vi "Model Initial Values - Model On Delete Action.vi"(6 "All deleted Refs":T1[](array[typedef]) format="%.0x", 8 "error in (no error)":errorcluster, 11 "Item Ref in":T1 format="%.0x") -> (0 "error out":errorcluster, 3 "Item Ref out":T1 format="%.0x")   [LabVIEW 2011, in "Model Initial Values Custom Device.lvlib"]
uses:
  Model Initial Values Custom Device.lvlib
  <vilib>/NI Veristand/Custom Device API/Custom Device Item Ref.ctl
  Model Initial Values - Global.vi
  <vilib>/NI Veristand/Custom Device API/Custom Device API.lvlib
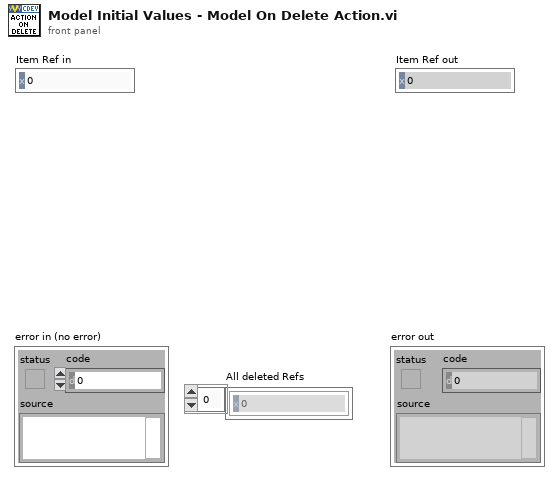
[diagram p1: front panel]
types:
  T1 = typedef "Custom Device API.lvlib/Custom Device Item Ref.ctl" = u64
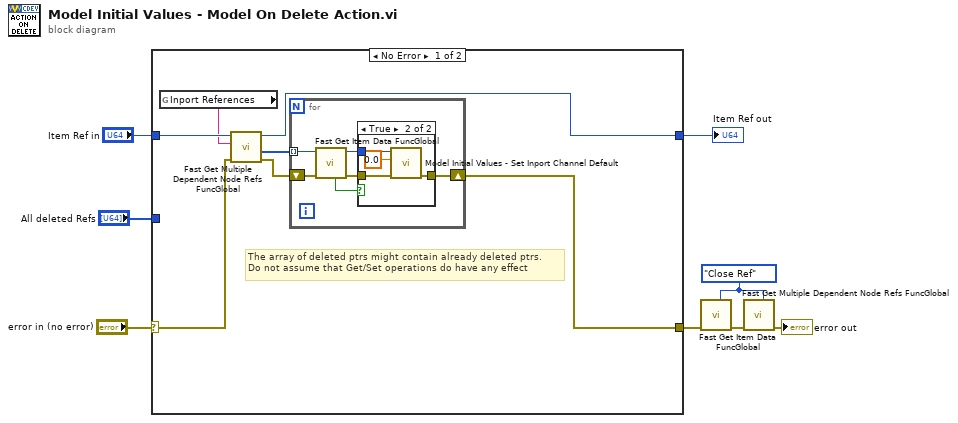
[diagram p0: block diagram]
diagram:
  w1 = enum16{"Open or Add", "Close Ref"}."Close Ref" ("Action")
  n1 = case shown="No Error" "error in (no error)" {
    selector: "error in (no error)" -> [w13 w28]
    tunnel: [w9 w28] -> w4
    tunnel: "Item Ref in" -> [w15 w27]
    tunnel: [w10 w27] -> w6
    tunnel: "All deleted Refs" -> [_ _]
    frame No Error {
      # "The array of deleted ptrs might contain already deleted ptrs.\nDo not assume that Get/Set operations do have any effect"
      n2 = global read "Model Initial Values - Global.vi" "Inport References"() -> (w14:string)
      n3 = call "Fast Get Multiple Dependent Node Refs FuncGlobal.vi"("error in (no error)"=w13, "Base Property Name"=w14, "Item Ref in"=w15) -> ("error out"=w11:errorcluster, "Dependent Node Refs"=w12:T1[], "Item Ref out"=w10:T1)  [unwired: 6 in]
      n4 = for {
        tunnel: w12 -> [w19] mode=indexing
        shift-right: [w21] -> w9
        shift-left: w11 -> [w20]
        n5 = call "Fast Get Item Data FuncGlobal.vi"("error in (no error)"=w20, "Item Ref in"=w19) -> ("error out"=w18:errorcluster, "Item Ref out"=w17:T1, "Found"=w16:bool)  [unwired: 6 in, 1 out]
        n6 = case shown="True" w16 {
          tunnel: [w22 w25] -> w21
          tunnel: w18 -> [w22 w24]
          tunnel: w17 -> [_ w23]
          frame False {
          }
          frame True {
            n7 = call "Model Initial Values - Set Inport Channel Default.vi"("error in"=w24, "Default Value"=0.0, "Item Ref in"=w23) -> ("error out"=w25:errorcluster)  [unwired: 7 in, 1 out]
          }
        }
      }
    }
    frame Error {
    }
  }
  "Item Ref out" <- w6
  n8 = call "Fast Get Item Data FuncGlobal.vi"("Action"=w1, "error in (no error)"=w4) -> ("error out"=w3:errorcluster)  [unwired: 6 in, 3 out]
  n9 = call "Fast Get Multiple Dependent Node Refs FuncGlobal.vi"("Action"=w1, "error in (no error)"=w3) -> ("error out"=→"error out":errorcluster)  [unwired: 7 in, 2 out]
